vi "DSF.Execution.Runtime.Plugin Manager.Name to Path.vi"(8 "error in (no error)":errorcluster, 10 "Plugin name":string, 11 "Plugin Manager in":refnum<class "DSF.Engine.Runtime.Plugin Manager.lvclass">) -> (0 "error out":errorcluster, 2 "Plugin folder":path, 3 "Plugin Manager out":refnum<class "DSF.Engine.Runtime.Plugin Manager.lvclass">)   [LabVIEW 2016, in "DSF.Engine.lvlib" / "DSF.Engine.Runtime.Plugin Manager.lvclass"]
uses:
  DSF.Engine.Runtime.Plugin Manager.lvclass
  DSF.Engine.Runtime.Plugin Manager.lvclass/DSF.Engine.Runtime.Plugin Manager.ctl
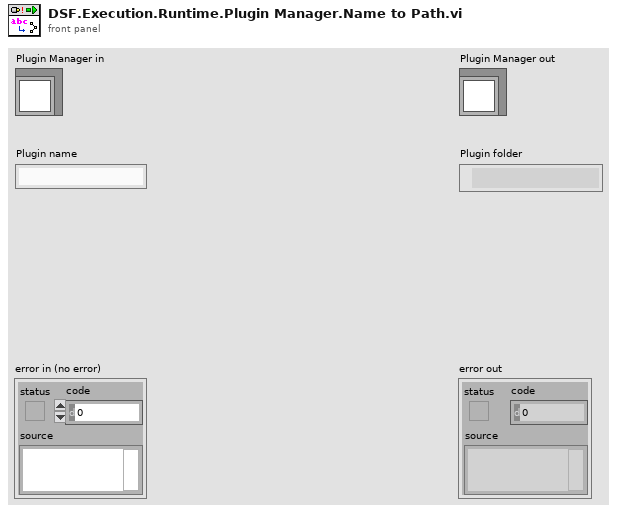
[diagram p1: front panel]
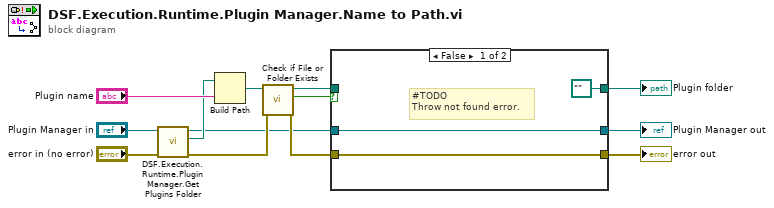
[diagram p0: block diagram]
diagram:
  n1 = call "DSF.Execution.Runtime.Plugin Manager.Get Plugins Folder.vi"("error in (no error)"="error in (no error)", "Plugin Manager in"="Plugin Manager in") -> ("error out"=w10:errorcluster, "Plugins folder"=w8:path, "Plugin Manager out"=w4:refnum<class "DSF.Engine.Runtime.Plugin Manager.lvclass">)  [unwired: 7 in]
  n2 = Build Path(base path=w8, name or relative path="Plugin name") -> (appended path=w11:path)
  n3 = call <vilib>:"Check if File or Folder Exists.vi"("error in (no error)"=w10, "path"=w11) -> ("error out"=w5:errorcluster, "file or folder exists?"=w7:bool, "dup path"=w2:path)  [unwired: 7 in]
  n4 = case shown="False" w7 {
    tunnel: [w15 w19] -> w6
    tunnel: w5 -> [w15 w19]
    tunnel: w4 -> [w16 w18]
    tunnel: [w16 w18] -> w3
    tunnel: w2 -> [_ w17]
    tunnel: [path "" ("dup path") w17] -> w1
    frame False {
      # "#TODO\nThrow not found error."
    }
    frame True {
    }
  }
  "error out" <- w6
  "Plugin Manager out" <- w3
  "Plugin folder" <- w1
